vi "UDP.Rx.Launch.vi"(5 "max size (548)":i32, 7 "port":u16, 8 "error in (no error)":errorcluster, 11 "Stop Pointer":refnum<class "Memory.Pointer.lvclass">) -> (0 "error out":errorcluster, 3 "Count Pointer":refnum<class "Memory.Pointer.lvclass">)   [LabVIEW 2017]
uses:
  <vilib>/National Instruments/Memory Manager/Classes/Pointer/Memory.Pointer.lvclass
  <vilib>/National Instruments/Memory Manager/Classes/Pointer/Memory.Pointer.lvclass/Memory.Pointer.ctl
  <vilib>/National Instruments/Memory Manager/Classes/Pointer/Memory.Pointer.New.4B.vi
  <vilib>/National Instruments/Memory Manager/Classes/Pointer/Memory.Pointer.Allocate.vi
  <vilib>/National Instruments/Memory Manager/Classes/Pointer/Memory.Pointer.Set Address.vi
  <vilib>/National Instruments/Memory Manager/Classes/Pointer/Memory.Pointer.Set Size.vi
  <vilib>/National Instruments/Memory Manager/Classes/Pointer/Memory.Pointer.Set Allocated.vi
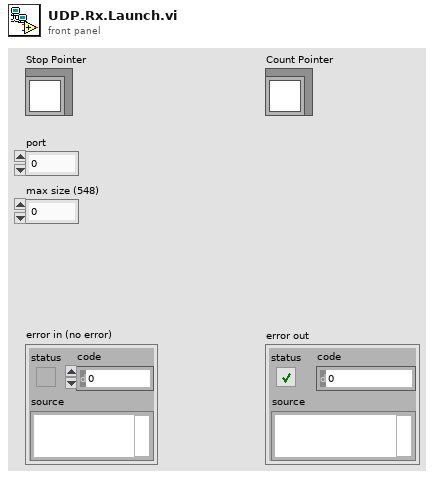
[diagram p1: front panel]
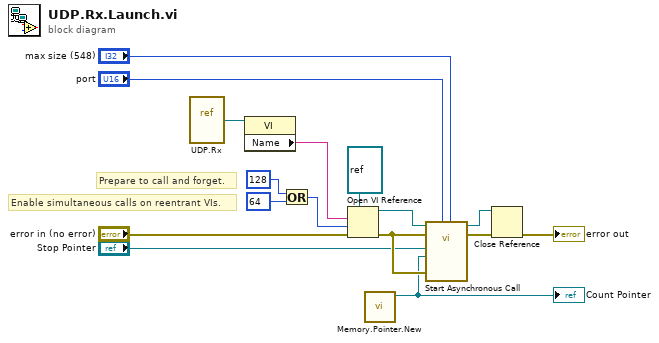
[diagram p0: block diagram]
diagram:
  # "Prepare to call and forget."
  # "Enable simultaneous calls on reentrant VIs."
  n1 = vi-ref "UDP.Rx.vi"() -> (w6:refnum<vi>)
  n2 = property class="VI"(reference=w6) -> ("Name"=w7:string)  [unwired: 1 in, 2 out]
  n3 = Or(x=128 ("options"), y=64 ("options")) -> (x .or. y?=w9:i32)
  n4 = Open VI Reference(type specifier VI Refnum (for type only)=refnum<vi> refnum, vi path=w7, options=w9, error in (no error)="error in (no error)") -> (vi reference=w14:refnum<vi>, error out=w16:errorcluster)  [unwired: 2 in]
  n5 = call-poly <vilib>:"Memory.Pointer.New.vi"() -> ("Pointer"=w1:refnum<class "Memory.Pointer.lvclass">)  [unwired: 10 in, 1 out]
  "Count Pointer" <- w1
  n6 = call-by-ref "Start Asynchronous Call"(reference=w14, error in=w16, "max size (548)"="max size (548)", "port"="port", 8:"error in (no error)"=w16, "Count Pointer"=w1, "Stop Pointer"="Stop Pointer") -> (reference out=w12:refnum<vi>, error out=w13:errorcluster)  [unwired: 6 in, 1 out]
  n7 = Close Reference(reference=w12, error in (no error)=w13) -> (error out=→"error out":errorcluster)
